vi "BB_Compute_Distance_fixed.vi"(8 "Y Image Resolution":i32, 9 "X Image Resolution":i32, 10 "Particle Scores":T1, 11 "Camera Type":enum16{"206", "1011"}(ring)) -> (1 "targetType":enum16{"Center", "Side", "Vertical"}(ring), 2 "Target Center (-1 to 1)":cluster{"X":dbl, "Y":dbl}, 3 "Distance (ft)":dbl)   [LabVIEW 2015]
doc: "Using the camera lens information and the real world size of the target, use trig and simple math to determine the distance to the target. Also returns the location relative to the image center in a (-1 , 1) coordinate system that may be useful for steering the robot."
panel:
  # "Axis 206\nAxis M1011"
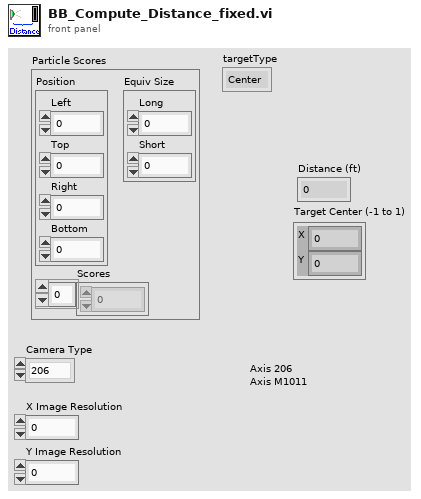
[diagram p1: front panel]
types:
  T1 = cluster{"Position":cluster{"Left":dbl, "Top":dbl, "Right":dbl, "Bottom":dbl}, "Scores":dbl[], "Equiv Size":cluster{"Long":dbl, "Short":dbl}}
  T2 = cluster{"X Image Resolution":i32, "Y Image Resolution":i32}
  T3 = cluster{"X Image Resolution":dbl, "Y Image Resolution":dbl}
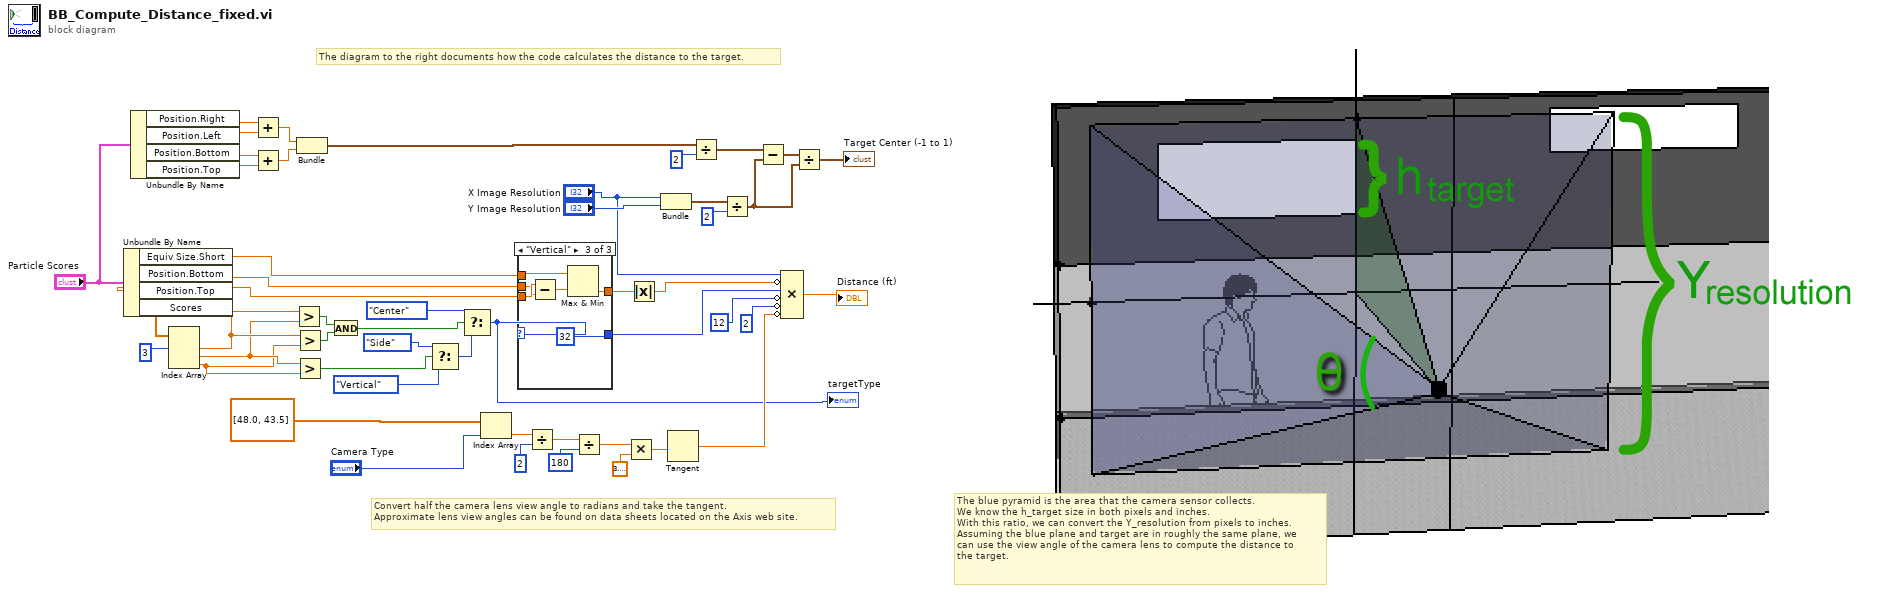
[diagram p0: block diagram]
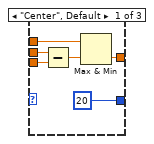
[diagram p2: hidden frame]
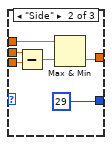
[diagram p3: hidden frame]
diagram:
  # "The blue pyramid is the area that the camera sensor collects.\nWe know the h_target size in both pixels and inches.\nWith this ratio, we can convert the Y_resolution from pixels to inches.\nAssuming the blue plane and target are in roughly the same plane, we\ncan use the view angle of the camera lens to compute the distance to\nthe target."
  # "Convert half the camera lens view angle to radians and take the tangent.\nApproximate lens view angles can be found on data sheets located on the Axis web site."
  # "The diagram to the right documents how the code calculates the distance to the target."
  n1 = Unbundle By Name("Particle Scores") -> ("Equiv Size.Short"=w6:dbl, "Position.Bottom"=w4:dbl, "Position.Top"=w3:dbl, "Scores"=w20:dbl[])
  n2 = Unbundle By Name("Particle Scores") -> ("Position.Right"=w38:dbl, "Position.Left"=w39:dbl, "Position.Bottom"=w41:dbl, "Position.Top"=w40:dbl)
  n3 = Index Array(array=w20, index #1=3) -> (element #1=w19:dbl, element #2=w12:dbl, element #3=w11:dbl)  [unwired: 2 in]
  n4 = Add(x=w38, y=w39) -> (x+y=w36:dbl)
  n5 = Add(x=w41, y=w40) -> (x+y=w35:dbl)
  n6 = Greater?(x=w19, y=w12) -> (0:w17:bool)
  n7 = Greater?(x=w19, y=w11) -> (0:w18:bool)
  n8 = Greater?(x=w12, y=w11) -> (0:w10:bool)
  n9 = Bundle(w36, w35) -> (w32:cluster{dbl, dbl})  [unwired: 1 in]
  n10 = And(x=w17, y=w18) -> (x .and. y?=w16:bool)
  n11 = Select(t=enum16{"Center", "Side", "Vertical"}."Side" ("targetType"), s=w10, f=enum16{"Center", "Side", "Vertical"}."Vertical" ("targetType")) -> (s? t:f=w14:enum16{"Center", "Side", "Vertical"})
  n12 = Select(t=enum16{"Center", "Side", "Vertical"}."Center" ("targetType"), s=w16, f=w14) -> (s? t:f=w8:enum16{"Center", "Side", "Vertical"})
  "targetType" <- w8
  n13 = Index Array(array=dbl[] [48.0, 43.5], index="Camera Type") -> (element=w48:dbl)
  n14 = case shown="\"Vertical\"" w8 {
    tunnel: [20 ("Target Height (in)") 29 ("Target Height (in)") 32 ("Target Height (in)")] -> w7
    tunnel: w6 -> [w54 w58 w66]
    tunnel: [w53 w57 w67] -> w5
    tunnel: w4 -> [w52 w61 w64]
    tunnel: w3 -> [w51 w60 w65]
    frame "Center", Default {
      n15 = Subtract(x=w52, y=w51) -> (x-y=w55:dbl)
      n16 = Max & Min(x=w54, y=w55) -> (min(x,y)=w53:dbl)  [unwired: 1 out]
    }
    frame "Side" {
      n17 = Subtract(x=w61, y=w60) -> (x-y=w59:dbl)
      n18 = Max & Min(x=w58, y=w59) -> (min(x,y)=w57:dbl)  [unwired: 1 out]
    }
    frame "Vertical" {
      n19 = Subtract(x=w65, y=w64) -> (x-y=w63:dbl)
      n20 = Max & Min(x=w66, y=w63) -> (min(x,y)=w67:dbl)  [unwired: 1 out]
    }
  }
  n21 = Divide(x=w48, y=2) -> (x/y=w45:dbl)
  n22 = Divide(x=w45, y=180) -> (x/y=w44:dbl)
  n23 = Multiply(x=w44, y=3.141592653589793) -> (x*y=w46:dbl)
  n24 = Absolute Value(x=w5) -> (abs(x)=w2:dbl)
  n25 = Bundle("X Image Resolution"="X Image Resolution", "Y Image Resolution"="Y Image Resolution") -> (w34:T2)  [unwired: 1 in]
  n26 = Tangent(1:w46) -> (0:w25:dbl)
  n27 = Divide(x=w32, y=2) -> (x/y=w31:cluster{dbl, dbl})
  n28 = Divide(x=w34, y=2) -> (x/y=w29:T3)
  n29 = Subtract(x=w31, y=w29) -> (x-y=w30:cluster{dbl, dbl})
  n30 = Compound Arithmetic op=MULTIPLY("X Image Resolution", invert w2, w7, invert 12, invert 2, invert w25) -> (→"Distance (ft)":dbl)
  n31 = Divide(x=w30, y=w29) -> (x/y=→"Target Center (-1 to 1)":cluster{dbl, dbl})
